vi "ClimbControlLoop.vi"   [LabVIEW 2018]
uses:
  <vilib>/Rock Robotics/WPI/Solenoid/WPI_SolenoidChannel.ctl
  <vilib>/Rock Robotics/WPI/SafetyOutput/WPI_SafetyOutputConfigMenu.ctl
  <vilib>/Rock Robotics/WPI/Solenoid/WPI_SolenoidOpenDouble.vi
  Robot Global Data.vi
  <vilib>/Rock Robotics/WPI/Solenoid/WPI_SolenoidSetEnum.vi
  Infrastructure/RobotMap.vi
  <vilib>/Rock Robotics/WPI/ThirdParty/Phoenix-LabVIEW/Motor Controller/Controls/CTRE_Phoenix_MotorControl_NeutralMode.ctl
  <vilib>/Rock Robotics/WPI/ThirdParty/Phoenix-LabVIEW/Motor Controller/Controls/CTRE_Phoenix_MotorControl_ControlMode.ctl
  <vilib>/Rock Robotics/WPI/Switch/WPI_SwitchOpenLimit.vi
types:
  T1 = typedef "WPI_SafetyOutputConfigMenu.ctl" = enum16{"Enable", "Disable"}
  T2 = typedef "WPI_SolenoidChannel.ctl" = enum8{"Solenoid 0", "Solenoid 1", "Solenoid 2", "Solenoid 3", "Solenoid 4", "Solenoid 5", "Solenoid 6", "Solenoid 7", "Invalid"}
  T3 = typedef "CTRE_Phoenix_MotorControl_NeutralMode.ctl" = enum8{"EEPROMSetting", "Override to Coast", "Override to Brake"}
  T4 = enum16{"FollowerType_PercentOutput", "FollowerType_AuxOutput1"}
  T5 = typedef "FPGA_DIOChannel.ctl" = enum8{"DIO 0", "DIO 1", "DIO 2", "DIO 3", "DIO 4", "DIO 5", "DIO 6", "DIO 7", "DIO 8", "DIO 9", "DIO MXP 0", "DIO MXP 1", "DIO MXP 2", "DIO MXP 3", "DIO MXP 4", "DIO MXP 5", "DIO MXP 6", "DIO MXP 7", "DIO MXP 8", "DIO MXP 9", "DIO MXP 10", "DIO MXP 11", "DIO MXP 12", "DIO MXP 13", "DIO MXP 14", "DIO MXP 15", "SPI Port CS1", "SPI Port CS2", "SPI Port CS3", "SPI Port MISO", "SPI Port MOSI", "Invalid"}
  T6 = typedef "WPI_MotorControlDeviceRef.ctl" = cluster{"DeviceStatus":errorcluster, "Type":T7, "PWM":cluster{"PWM Channel":T8, "DeadBand":T9}, "CAN":cluster{"Device Number":u8, "SetOutput VI Ref":variant, "GetOutput VI Ref":variant, "Enable VI Ref":variant, "Disable VI Ref":variant, "Data":variant}, "Invert":bool, "DIO PWM":cluster{"PWM \"Enable\" Channel":T8, "DIOChannel":T5, "PWM Rate":dbl}}
  T7 = typedef "WPI_MotorControlType.ctl" = enum16{"PWM", "CAN", "DIO PWM"}
  T8 = typedef "FPGA_DIOPWMChannel.ctl" = enum8{"PWM 0", "PWM 1", "PWM 2", "PWM 3", "PWM 4", "PWM 5", "PWM 6", "PWM 7", "PWM 8", "PWM 9", "PWM MXP 0", "PWM MXP 1", "PWM MXP 2", "PWM MXP 3", "PWM MXP 4", "PWM MXP 5", "PWM MXP 6", "PWM MXP 7", "PWM MXP 8", "PWM MXP 9", "Invalid"}
  T9 = typedef "WPI_PWMDeadband.ctl" = cluster{"Name":string, "maxPositivePwm":i32, "minPositivePwm":i32, "centerPwm":i32, "maxNegativePwm":i32, "minNegativePwm":i32, "angularRange":u16}
  T10 = typedef "WPI_SwitchDevRef.ctl" = cluster{"DevStatus":errorcluster, "DIO Channel":T5, "CntIndex":T11, "Normally Closed":bool}
  T11 = typedef "FPGA_CounterCtrSystemIndex.ctl" = enum8{"Ctr 0", "Ctr 1", "Ctr 2", "Ctr 3", "Ctr 4", "Ctr 5", "Ctr 6", "Ctr 7", "Invalid"}
  T12 = typedef "WPI_JoystickDevRef.ctl" = cluster{"Device":T13}
  T13 = typedef "WPI_JoystickDeviceEnum.ctl" = enum16{"USB 0", "USB 1", "USB 2", "USB 3", "USB 4", "USB 5"}
  T14 = typedef "CTRE_Phoenix_MotorControl_ControlMode.ctl" = u16
  T15 = typedef "WPI_SolenoidDevRef.ctl" = cluster{"DevStatus":errorcluster, "Pneumatics Control Module":u8, "Forward Solenoid Channel":T2, "Reverse Solenoid Channel":T2}
  T16 = typedef "WPI_SolenoidValue.ctl" = enum16{"Off", "On", "Forward", "Reverse"}
  T17 = cluster{"Front Climb Output":T16, "Rear Climb Output":T16}
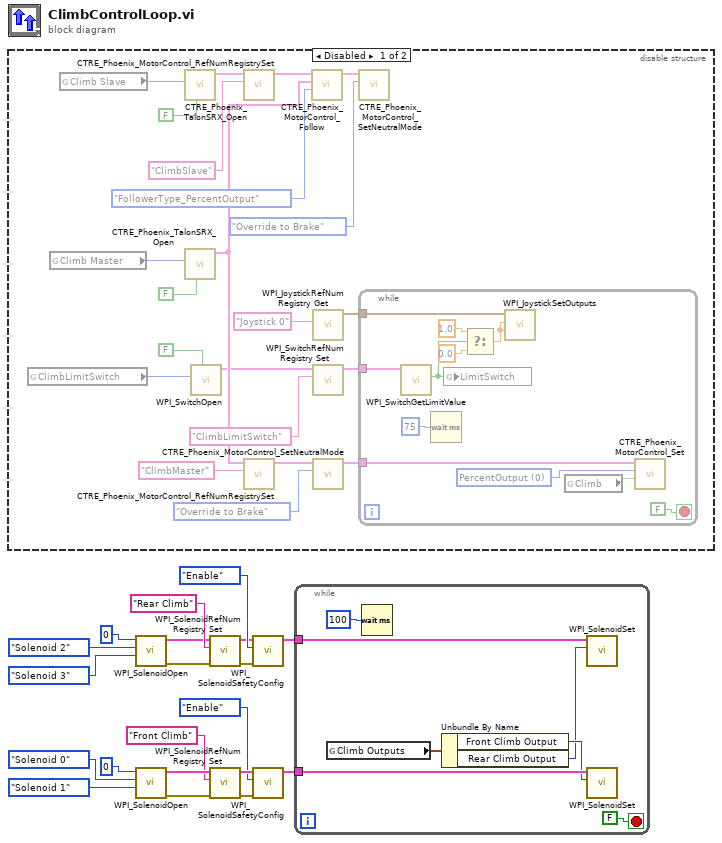
[diagram p0: block diagram]
diagram:
  n1 = disable-structure shown="Disabled" {
    frame Disabled {
      n2 = global read "RobotMap.vi" "ClimbLimitSwitch"() -> (w28:T5)
      n3 = global read "RobotMap.vi" "Climb Master"() -> (w42:u8)
      n4 = global read "RobotMap.vi" "Climb Slave"() -> (w41:u8)
      n5 = call <vilib>:"CTRE_Phoenix_TalonSRX_Open.vi"("Invert"=FALSE, "Device Number"=w41) -> ("CAN Talon SRX Ref"=w40:T6)  [unwired: 8 in, 1 out]
      n6 = call <vilib>:"CTRE_Phoenix_TalonSRX_Open.vi"("Invert"=FALSE, "Device Number"=w42) -> ("CAN Talon SRX Ref"=w39:T6)  [unwired: 8 in, 1 out]
      n7 = call-poly <vilib>:"WPI_SwitchOpen.vi"("Normally Closed"=FALSE, "DIO Channel"=w28) -> ("SwitchDevRef"=w27:T10)  [unwired: 8 in, 1 out]
      n8 = call <vilib>:"CTRE_Phoenix_MotorControl_RefNumRegistrySet.vi"("refnum name"="ClimbSlave", "PhoenixMotorControlDevRef"=w40) -> ("PhoenixMotorControlDevRef"=w38:T6)  [unwired: 8 in, 1 out]
      n9 = call <vilib>:"CTRE_Phoenix_MotorControl_RefNumRegistrySet.vi"("refnum name"="ClimbMaster", "PhoenixMotorControlDevRef"=w39) -> ("PhoenixMotorControlDevRef"=w30:T6)  [unwired: 8 in, 1 out]
      n10 = call <vilib>:"CTRE_Phoenix_MotorControl_Follow.vi"("FollowerType"=T4."FollowerType_PercentOutput", "Master Controller to Follow"=w39, "PhoenixMotorControlDevRef"=w38) -> ("PhoenixMotorControlDevRef"=w32:T6)  [unwired: 7 in, 1 out]
      n11 = call <vilib>:"WPI_JoystickRefNum Registry Get.vi"("refnum name"="Joystick 0") -> ("JoystickDevRef"=w21:T12)  [unwired: 1 in, 9 out]
      n12 = call <vilib>:"WPI_SwitchRefNum Registry Set.vi"("refnum name"="ClimbLimitSwitch", "SwitchDevRef"=w27) -> ("SwitchDevRef"=w26:T10)  [unwired: 8 in, 1 out]
      n13 = call <vilib>:"CTRE_Phoenix_MotorControl_SetNeutralMode.vi"("Motor Control Neutral Mode"=CTRE_Phoenix_MotorControl_NeutralMode."Override to Brake", "PhoenixMotorControlDevRef"=w30) -> ("PhoenixMotorControlDevRef"=w22:T6)  [unwired: 8 in, 1 out]
      n14 = call <vilib>:"CTRE_Phoenix_MotorControl_SetNeutralMode.vi"("Motor Control Neutral Mode"=CTRE_Phoenix_MotorControl_NeutralMode."Override to Brake", "PhoenixMotorControlDevRef"=w32) -> ()  [unwired: 8 in, 2 out]
      n15 = while {
        tunnel: w26 -> [w52]
        tunnel: w22 -> [w48]
        tunnel: w21 -> [w45]
        stop <- FALSE stop-if-true
        w53 = T14 0 items=["PercentOutput"=0, "Position"=1, "Velocity"=2, "Current"=3, "Follower"=5, "MotionProfile"=6, "MotionMagic"=7, "MotionProfileArc"=10, "Disabled"=15] ("Control Mode")
        n16 = call <vilib>:"WPI_SwitchGetLimitValue.vi"("SwitchDevRef"=w52) -> ("Switch Pressed"=w44:bool)  [unwired: 8 in, 2 out]
        n17 = Wait (ms)(milliseconds to wait=u32 75) -> ()  [unwired: 1 out]
        n18 = global write "Robot Global Data.vi" "LimitSwitch"(w44) -> ()
        n19 = Select(t=sgl 1.0 ("Left Rumble"), s=w44, f=sgl 0.0) -> (s? t:f=w47:sgl)
        n20 = call <vilib>:"WPI_JoystickSetOutputs.vi"("Right Rumble"=w47, "Left Rumble"=w47, "JoystickDevRef"=w45) -> ()  [unwired: 7 in, 2 out]
        n21 = global read "Robot Global Data.vi" "Climb"() -> (w51)
        n22 = call <vilib>:"CTRE_Phoenix_MotorControl_Set.vi"("Output"=w51, "Control Mode"=w53, "PhoenixMotorControlDevRef"=w48) -> ()  [unwired: 7 in, 2 out]
      }
    }
    frame Enabled {
    }
  }
  n23 = call-poly <vilib>:"WPI_SolenoidOpen.vi"("Reverse Solenoid Channel"=WPI_SolenoidChannel."Solenoid 3", "Forward Solenoid Channel"=WPI_SolenoidChannel."Solenoid 2", "Pneumatics Control Module (0)"=u8 0) -> ("error out"=w6:errorcluster, "SolenoidDevRef"=w7:T15)  [unwired: 7 in]
  n24 = call-poly <vilib>:"WPI_SolenoidOpen.vi"("Reverse Solenoid Channel"=WPI_SolenoidChannel."Solenoid 1", "Forward Solenoid Channel"=WPI_SolenoidChannel."Solenoid 0", "Pneumatics Control Module (0)"=u8 0) -> ("error out"=w17:errorcluster, "SolenoidDevRef"=w16:T15)  [unwired: 7 in]
  n25 = call <vilib>:"WPI_SolenoidRefNum Registry Set.vi"("error in (no error)"=w6, "refnum name"="Rear Climb", "SolenoidDevRef"=w7) -> ("error out"=w8:errorcluster, "SolenoidDevRef"=w9:T15)  [unwired: 7 in]
  n26 = call <vilib>:"WPI_SolenoidRefNum Registry Set.vi"("error in (no error)"=w17, "refnum name"="Front Climb", "SolenoidDevRef"=w16) -> ("error out"=w15:errorcluster, "SolenoidDevRef"=w14:T15)  [unwired: 7 in]
  n27 = call <vilib>:"WPI_SolenoidSafetyConfig.vi"("error in (no error)"=w8, "mode"=WPI_SafetyOutputConfigMenu."Enable", "SolenoidDevRef"=w9) -> ("SolenoidDevRef"=w1:T15)  [unwired: 7 in, 1 out]
  n28 = call <vilib>:"WPI_SolenoidSafetyConfig.vi"("error in (no error)"=w15, "mode"=WPI_SafetyOutputConfigMenu."Enable", "SolenoidDevRef"=w14) -> ("SolenoidDevRef"=w2:T15)  [unwired: 7 in, 1 out]
  n29 = while {
    tunnel: w2 -> [w60]
    tunnel: w1 -> [w59]
    stop <- FALSE stop-if-true
    n30 = global read "Robot Global Data.vi" "Climb Outputs"() -> (w58:T17)
    n31 = Wait (ms)(milliseconds to wait=u32 100) -> ()  [unwired: 1 out]
    n32 = Unbundle By Name(w58) -> ("Front Climb Output"=w57:T16, "Rear Climb Output"=w56:T16)
    n33 = call-poly <vilib>:"WPI_SolenoidSet.vi"("Value"=w56, "SolenoidDevRef"=w59) -> ()  [unwired: 8 in, 2 out]
    n34 = call-poly <vilib>:"WPI_SolenoidSet.vi"("Value"=w57, "SolenoidDevRef"=w60) -> ()  [unwired: 8 in, 2 out]
  }
